vi "Configure SLSC Switch Custom Device.vi"(6 "model":string, 7 "resource":string, 8 "error in (no error)":errorcluster, 9 "switches json":string, 10 "topologies":string[](array[string]), 11 "SLSC Switch Custom Device Ref in":T1 format="%.0x") -> (0 "error out":errorcluster, 3 "SLSC Switch Custom Device Ref out":T1 format="%.0x")   [LabVIEW 2017, in "SLSC Switch Scripting.lvlib"]
uses:
  SLSC Switch Scripting.lvlib
  <vilib>/NI Veristand/Custom Device API/Custom Device Item Ref.ctl
  Properties/SLSC Switch All Properties.ctl
  Shared/Routing and Faulting Hardware API/Routing and Faulting Hardware API.lvlib
  <vilib>/NI Veristand/Custom Device API/Custom Device API.lvlib
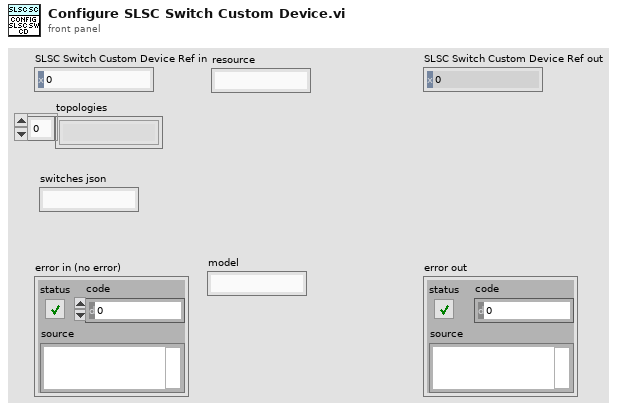
[diagram p1: front panel]
types:
  T1 = typedef "Custom Device API.lvlib/Custom Device Item Ref.ctl" = u64
  T2 = typedef "SLSC Switch Scripting.lvlib/SLSC Switch All Properties.ctl" = cluster{"Model":string, "Resource":string, "Topology":string, "Capabilities":string, "Description":string}
  T3 = typedef "Routing and Faulting Hardware API.lvlib/Possible Connections for Endpoint.ctl" = cluster{"Source":string, "Destinations":string[]}
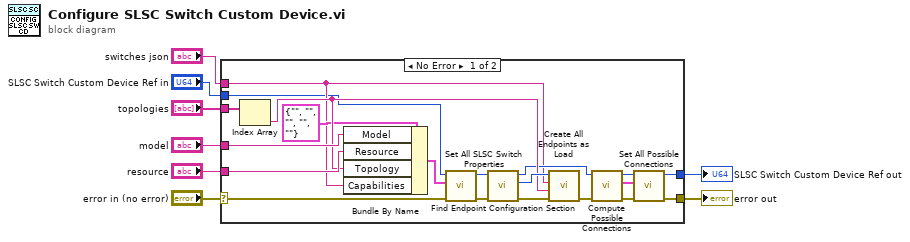
[diagram p0: block diagram]
diagram:
  n1 = case shown="No Error" "error in (no error)" {
    selector: "error in (no error)" -> [w9 w29]
    tunnel: "model" -> [w28 _]
    tunnel: "resource" -> [w27 _]
    tunnel: [w17 w29] -> w6
    tunnel: [w16 w30] -> w5
    tunnel: "topologies" -> [w12 _]
    tunnel: "switches json" -> [w11 _]
    tunnel: "SLSC Switch Custom Device Ref in" -> [w10 w30]
    frame No Error {
      n2 = Index Array(array=w12) -> (element=w23:string)  [unwired: 1 in]
      n3 = Bundle By Name(cluster=T2 {"Model"="", "Resource"="", "Topology"="", "Capabilities"="", "Description"=""} ("SLSC Switch All Properties"), "Model"=w28, "Resource"=w27, "Topology"=w23, "Capabilities"=w11) -> (w13:T2)
      n4 = call "Set All SLSC Switch Properties.vi"("error in (no error)"=w9, "SLSC Switch All Properties"=w13, "SLSC Switch Custom Device Ref in"=w10) -> ("error out"=w26:errorcluster, "SLSC Switch Custom Device Ref out"=w15:T1)  [unwired: 7 in]
      n5 = call "Find Endpoint Configuration Section.vi"("error in (no error)"=w26, "SLSC Switch Custom Device Ref in"=w15) -> ("error out"=w25:errorcluster, "Endpoint Config Section Ref"=w24:T1, "SLSC Switch Custom Device Ref out"=w19:T1)  [unwired: 7 in]
      n6 = call "Create All Endpoints as Load.vi"("error in (no error)"=w25, "topology"=w23, "switches json"=w11, "Endpoint Config Section Ref"=w24) -> ("error out"=w18:errorcluster)  [unwired: 6 in, 1 out]
      n7 = call "Compute Possible Connections.vi"("error in (no error)"=w18, "Item Ref in"=w19) -> ("error out"=w21:errorcluster, "Possible Connections"=w22:T3[], "Item Ref out"=w20:T1)  [unwired: 7 in]
      n8 = call "Set All Possible Connections.vi"("error in (no error)"=w21, "Possible Connections"=w22, "Hardware Ref in"=w20) -> ("error out"=w17:errorcluster, "Hardware Ref out"=w16:T1)  [unwired: 7 in]
    }
    frame Error {
    }
  }
  "error out" <- w6
  "SLSC Switch Custom Device Ref out" <- w5
